vi "3.11-Filter Obstacle Data.vi"(1 "Obstacle Array":T1(array[cluster]), 2 "Y Array":dbl[](array[numeric]), 3 "X Array":dbl[](array[numeric])) -> (0 "output array":T1(array[cluster]))   [LabVIEW 2010]
uses:
  3.0-Global.vi
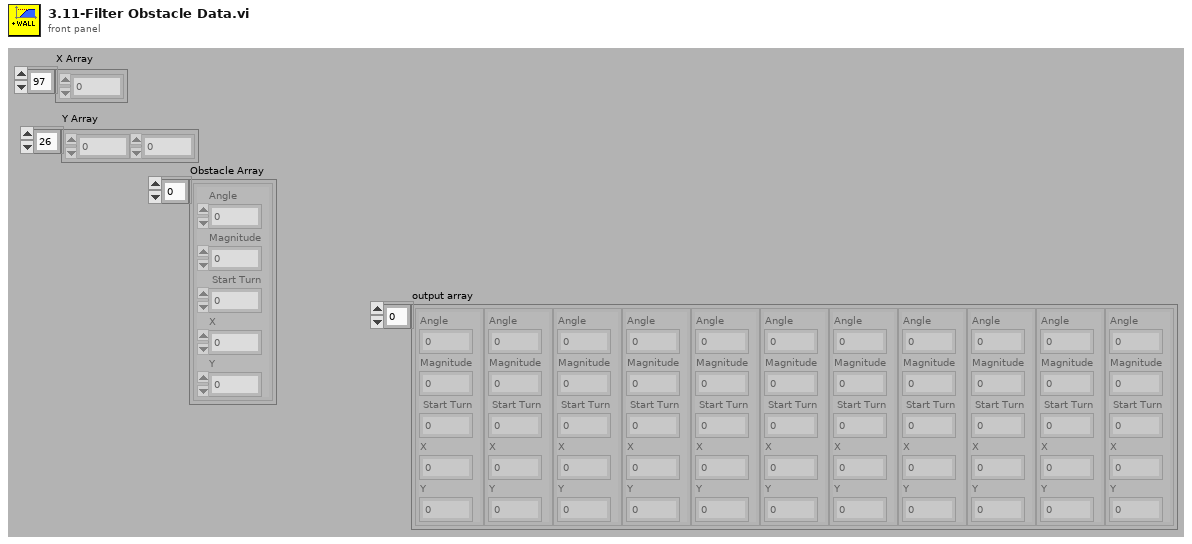
[diagram p1: front panel]
types:
  T1 = cluster{"Angle":dbl, "Magnitude":dbl, " Start Turn":dbl, "X":dbl, "Y":dbl}[]
  T2 = cluster{"Left Angle":dbl, "Left Magnitude":dbl, "Left Start Turn":dbl, "X":dbl, "Y":dbl}
  T3 = cluster{"Right Angle":dbl, "Right Magnitude":dbl, "Right Start Turn":dbl, "X":dbl, "Y":dbl}
  T4 = cluster{"Left Angle":dbl, "Left Magnitude":dbl, "Left Start Turn":dbl, "X":dbl, "Y":dbl}[]
  T5 = cluster{"Right Angle":dbl, "Right Magnitude":dbl, "Right Start Turn":dbl, "X":dbl, "Y":dbl}[]
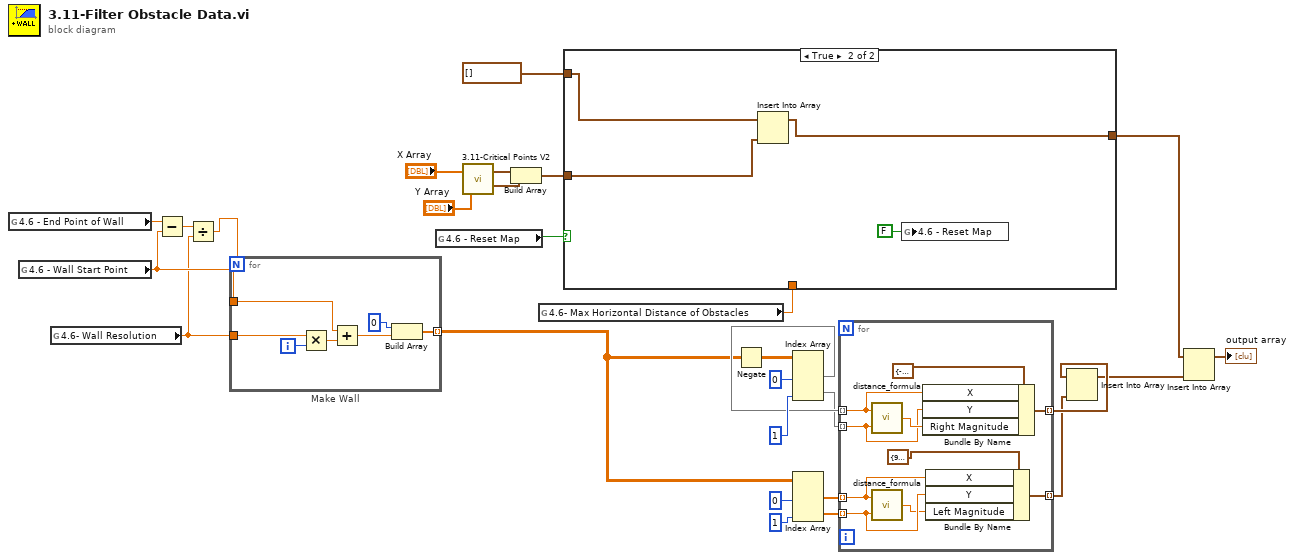
[diagram p0: block diagram]
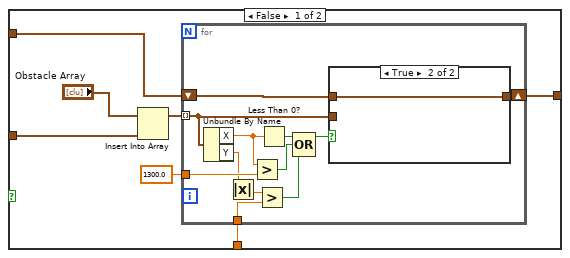
[diagram p2: hidden frame]
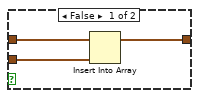
[diagram p3: hidden frame]
diagram:
  n1 = global read "3.0-Global.vi" "4.6 - End Point of Wall"() -> (w5:dbl)
  n2 = global read "3.0-Global.vi" "4.6 - Wall Start Point"() -> (w4:dbl)
  n3 = global read "3.0-Global.vi" "4.6- Wall Resolution"() -> (w3:dbl)
  n4 = Subtract(x=w5, y=w4) -> (x-y=w8:dbl)
  n5 = Divide(x=w8, y=w3) -> (x/y=w9:dbl)
  n6 = for "Make Wall" {
    N: w9 -> [_]
    tunnel: [w32] -> w6 mode=indexing
    tunnel: w3 -> [w31]
    tunnel: w4 -> [w29]
    i -> [w30]
    n7 = Multiply(x=w31, y=w30) -> (x*y=w35:dbl)
    n8 = Add(x=w29, y=w35) -> (x+y=w33:dbl)
    n9 = Build Array(0 ("x"), w33) -> (w32:dbl[])
  }
  n10 = global read "3.0-Global.vi" "4.6 - Reset Map"() -> (w1:bool)
  n11 = call "3.11-Critical Points V2.vi"("Y (mm)"="Y Array", "X (mm)"="X Array") -> ("Left Data"=w16:T2, "Right Data"=w17:T3)
  n12 = Build Array(w17, w16) -> (w15:T4)
  n13 = global read "3.0-Global.vi" "4.6- Max Horizontal Distance of Obstacles"() -> (w2:dbl)
  n14 = case shown="True" w1 {
    tunnel: [w42 w60] -> w18
    tunnel: w15 -> [w40 w61]
    tunnel: T1 [] ("Obstacle Array") -> [w39 w62]
    tunnel: w2 -> [w37 _]
    frame False {
      n15 = Insert Into Array(array="Obstacle Array", new element=w40) -> (w41:T1)  [unwired: 1 in]
      n16 = for {
        shift-right: [w53] -> w42
        shift-left: w39 -> [w54]
        tunnel: w41 -> [w52] mode=indexing
        tunnel: 1300.0 -> [w48]
        tunnel: w37 -> [w44]
        n17 = Unbundle By Name(w52) -> ("X"=w49:dbl, "Y"=w45:dbl)
        n18 = Absolute Value(x=w45) -> (abs(x)=w43:dbl)
        n19 = Greater?(x=w49, y=w48) -> (0:w47:bool)
        n20 = Greater?(x=w43, y=w44) -> (0:w46:bool)
        n21 = Less Than 0?(x=w49) -> (x < 0?=w50:bool)
        n22 = Compound Arithmetic op=OR(w50, w47, w46) -> (w51:bool)
        n23 = case shown="True" w51 {
          tunnel: w54 -> [w57 w58]
          tunnel: [w56 w58] -> w53
          tunnel: w52 -> [w55 _]
          frame False {
            n24 = Insert Into Array(array=w57, new element=w55) -> (w56:T1)  [unwired: 1 in]
          }
          frame True {
          }
        }
      }
    }
    frame True {
      n25 = Insert Into Array(array=w62, new element=w61) -> (w60:T1)  [unwired: 1 in]
      n26 = global write "3.0-Global.vi" "4.6 - Reset Map"(FALSE ("4.6 - Reset Map")) -> ()
    }
  }
  n27 = Negate(x=w6) -> (-x=w7:dbl[][])
  n28 = Index Array(array=w7, index (col) #1=0 ("disabled index (col)"), index (col) #2=1 ("index (col)")) -> (element #1=w22:dbl[], element #2=w21:dbl[])  [unwired: 2 in]
  n29 = Index Array(array=w6, index (col) #1=0 ("disabled index (col)"), index (col) #2=1 ("index (col)")) -> (element #1=w20:dbl[], element #2=w19:dbl[])  [unwired: 2 in]
  n30 = for {
    tunnel: w22 -> [w66] mode=indexing
    tunnel: w21 -> [w65] mode=indexing
    tunnel: w20 -> [w71] mode=indexing
    tunnel: w19 -> [w72] mode=indexing
    tunnel: [w64] -> w13 mode=indexing
    tunnel: [w63] -> w12 mode=indexing
    n31 = call "distance_formula.vi"("X2 - X1"=w65, "Y2 - Y1"=w66) -> ("Distance"=w67:dbl)
    n32 = call "distance_formula.vi"("X2 - X1"=w72, "Y2 - Y1"=w71) -> ("Distance"=w70:dbl)
    n33 = Bundle By Name(cluster=T3 {"Right Angle"=-90.0, "Right Magnitude"=0.0, "Right Start Turn"=-90.0, "X"=0.0, "Y"=0.0} ("Right Data"), "X"=w66, "Y"=w65, "Right Magnitude"=w67) -> (w64:T3)
    n34 = Bundle By Name(cluster=T2 {"Left Angle"=90.0, "Left Magnitude"=0.0, "Left Start Turn"=90.0, "X"=0.0, "Y"=0.0} ("Left Data"), "X"=w71, "Y"=w72, "Left Magnitude"=w70) -> (w63:T2)
  }
  n35 = Insert Into Array(array=w13, new element=w12) -> (w11:T5)  [unwired: 1 in]
  n36 = Insert Into Array(array=w18, new element=w11) -> (→"output array":T1)  [unwired: 1 in]
